vi "mux2-1(DMM I)_encode.vi"(8 "error in (no error)":errorcluster, 10 "mux2-1(DMM I)":enum16{"DMM I (0.5)", "DMM I (12)"}(ring)=enum."DMM I (12)", 11 "Mem_mapping in":u16[](array[numeric])) -> (0 "error out":errorcluster, 3 "MemMapping Out":u16[](array[numeric]))   [LabVIEW 2018, in "MB Relay.lvlib"]
uses:
  MB Relay.lvlib
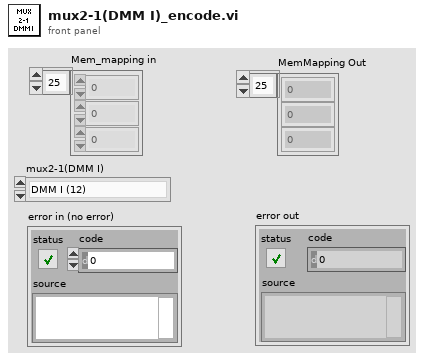
[diagram p1: front panel]
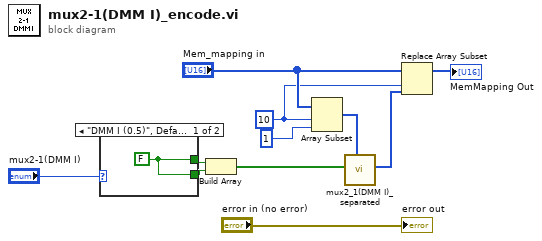
[diagram p0: block diagram]
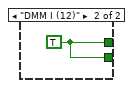
[diagram p2: hidden frame]
diagram:
  w7 = 10 ("index")
  n1 = case shown="\"DMM I (0.5)\", Default" "mux2-1(DMM I)" {
    tunnel: [w12 w13] -> w4
    tunnel: [w12 w13] -> w3
    frame "DMM I (0.5)", Default {
      w12 = FALSE
    }
    frame "DMM I (12)" {
      w13 = TRUE
    }
  }
  n2 = Build Array(w4, w3) -> (w2:bool[])
  n3 = Array Subset(array="Mem_mapping in", index=w7, length=1) -> (w6:u16[])
  n4 = call "mux2_1(DMM I)_separated.vi"("Boolean array"=w2, "Mem_mapping in"=w6) -> ("Mem_mapping out"=w1:u16[])  [unwired: 8 in]
  n5 = Replace Array Subset(array="Mem_mapping in", new element=w1, index=w7) -> (→"MemMapping Out":u16[])
  "error out" <- "error in (no error)"
